vi "yolo_img_overlay.vi"(4 "Font, Size & Style":T1, 5 "Distances":cluster{string, dbl}[](array[cluster]), 6 "Class names":string[](array[string]), 7 "Input image":T2, 8 "error in (no error)":errorcluster, 9 "Scores":dbl[](array[numeric]), 10 "Numbered classes":dbl[](array[numeric]), 11 "BBoxes [y_min, x_min, y_max, x_max]":dbl[][](array[numeric])) -> (0 "error out":errorcluster, 2 "Detected class names":string[](array[string]), 3 "Overlaid image":T2)   [LabVIEW 2019]
uses:
  <vilib>/vision/Image Controls.llb/IMAQ Image.ctl
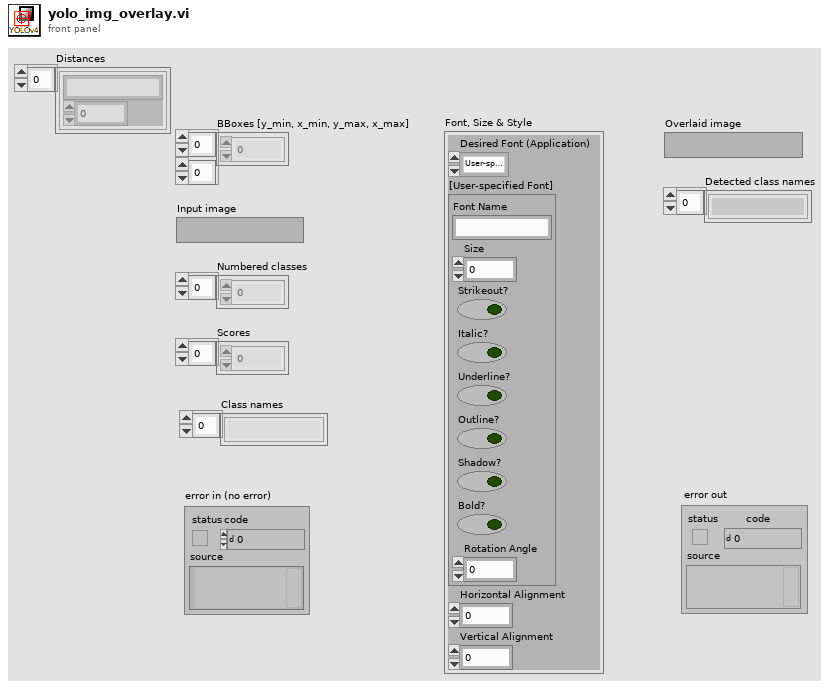
[diagram p1: front panel]
types:
  T1 = cluster{"Desired Font (Application)":enum16{"User-specified Font", "Application Font", "System Font", "Dialog Font"}, "[User-specified Font]":cluster{"Font Name":string, "Size":i16, "Strikeout?":bool, "Italic?":bool, "Underline?":bool, "Outline?":bool, "Shadow?":bool, "Bold?":bool, "Rotation Angle":dbl}, "Horizontal Alignment":i16, "Vertical Alignment":i16}
  T2 = typedef "IMAQ Image.ctl" = refnum<image>
  T3 = cluster{"[0]":dbl, "[1]":dbl, "[2]":dbl, "[3]":dbl}
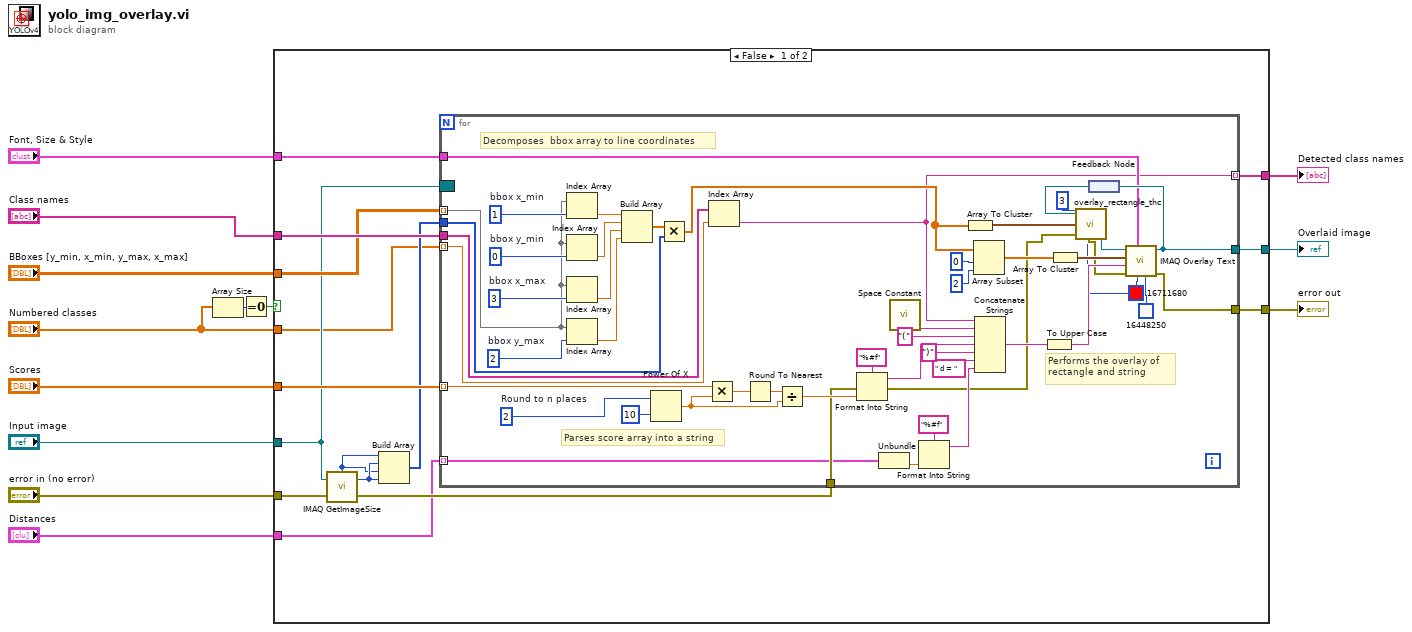
[diagram p0: block diagram]
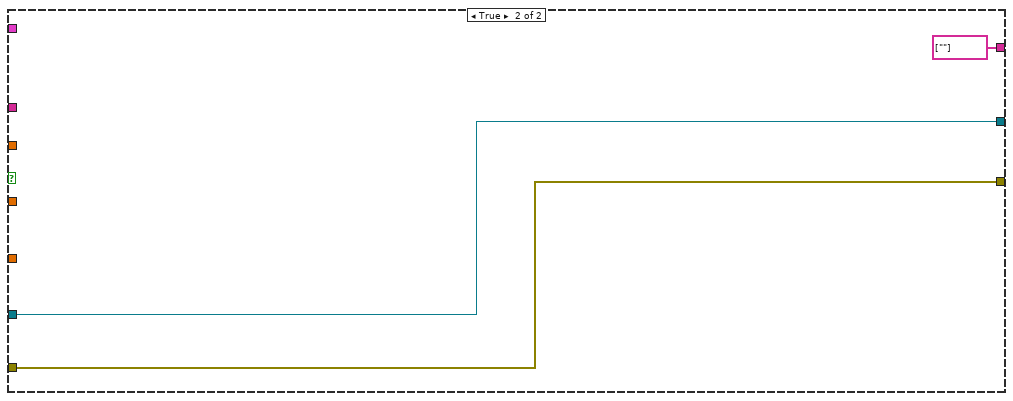
[diagram p2: hidden frame]
diagram:
  n1 = Array Size(array="Numbered classes") -> (size(s)=w4:i32)
  n2 = Equal To 0?(x=w4) -> (x = 0?=w2:bool)
  n3 = case shown="False" w2 {
    tunnel: [w28 w81] -> w13
    tunnel: "Class names" -> [w27 _]
    tunnel: "Scores" -> [w26 _]
    tunnel: [w22 string[] [""]] -> w10
    tunnel: "BBoxes [y_min, x_min, y_max, x_max]" -> [w21 _]
    tunnel: "Font, Size & Style" -> [w20 _]
    tunnel: "Input image" -> [w19 w81]
    tunnel: "error in (no error)" -> [w18 w80]
    tunnel: [w16 w80] -> w5
    tunnel: "Numbered classes" -> [w15 _]
    tunnel: "Distances" -> [w14 _]
    frame False {
      n4 = call "IMAQ GetImageSize"("Image"=w19, "error in (no error)"=w18) -> ("Y Resolution"=w25:i32, "X Resolution"=w24:i32, "error out"=w17:errorcluster)  [unwired: 2 in]
      n5 = Build Array(w24, w25, w24, w25) -> (w23:i32[])
      n6 = for {
        tunnel: w15 -> [w45] mode=indexing
        tunnel: w27 -> [w78]
        tunnel: [w47] -> w22 mode=indexing
        tunnel: w23 -> [w70]
        tunnel: [w69] -> w28
        tunnel: w26 -> [w54] mode=indexing
        tunnel: w20 -> [w48]
        tunnel: w21 -> [w46] mode=indexing
        border: w19 -> [_]
        tunnel: w17 -> [w44]
        tunnel: [w43] -> w16
        tunnel: w14 -> [w39] mode=indexing
        w31 = u32 16711680 ("Text Color (black)")
        w55 = 2  # Round to n places
        w75 = 3  # bbox x_max
        w74 = 2  # bbox y_max
        w73 = 1  # bbox x_min
        w72 = 0  # bbox y_min
        # "Performs the overlay of \nrectangle and string"
        # "Parses score array into a string"
        # "Decomposes  bbox array to line coordinates"
        n7 = Index Array(array=w46, index=w73) -> (element=w68:dbl)
        n8 = Index Array(array=w46, index=w72) -> (element=w67:dbl)
        n9 = Index Array(array=w46, index=w75) -> (element=w77:dbl)
        n10 = Index Array(array=w46, index=w74) -> (element=w76:dbl)
        n11 = Build Array(w68, w67, w77, w76) -> (w71:dbl[])
        n12 = Power Of X(1:10, 2:w55) -> (0:w51:dbl)
        n13 = Multiply(x=w71, y=w70) -> (x*y=w66:dbl[])
        n14 = Multiply(x=w54, y=w51) -> (x*y=w53:dbl)
        n15 = Index Array(array=w78, index=w45) -> (element=w47:string)
        n16 = Round To Nearest(number=w53) -> (nearest integer value=w52:dbl)
        n17 = Divide(x=w52, y=w51) -> (x/y=w50:dbl)
        n18 = Format Into String(format string="%#f", error in=w44, w50) -> (resulting string=w61:string, error out=w33:errorcluster)  [unwired: 1 in]
        n19 = Unbundle(w39) -> (w41:dbl)  [unwired: 1 out]
        n20 = call <vilib>:"Space Constant.vi"() -> ("String"=w42:string)
        n21 = Format Into String(format string="%#f", w41) -> (resulting string=w37:string)  [unwired: 2 in, 1 out]
        n22 = Array To Cluster(array=w66) -> (cluster=w29:T3)
        n23 = Array Subset(array=w66, index=0, length=2) -> (w63:dbl[])
        n24 = Concatenate Strings(w47, w42, "(" ("string"), w61, ")" ("string"), " d = " ("string"), w37) -> (w58:string)
        n25 = To Upper Case(1:w58) -> (0:w57:string)
        n26 = Array To Cluster(array=w63) -> (cluster=w62:cluster{"[0]":dbl, "[1]":dbl})
        n27 = feedback #1() -> (w35:T2)
        n28 = call "overlay_rectangle_thc.vi"("Image In"=w35, "Thickness"=3, "Rectangle"=w29, "Error In"=w33, "Color"=w31) -> ("Image Out"=w34:T2, "Error Out"=w32:errorcluster)
        n29 = call "IMAQ Overlay Text"("BG Color (Transparent)"=u32 16448250, "Text Color (black)"=w31, "Font, Size & Style"=w48, "error in (no error)"=w32, "String"=w57, "Origin"=w62, "Image"=w34) -> ("error out"=w43:errorcluster, "Image Out"=w69:T2)  [unwired: 3 in]
        n30 = feedback-in #1(w69) -> ()
      }
    }
    frame True {
    }
  }
  "Overlaid image" <- w13
  "Detected class names" <- w10
  "error out" <- w5
